vi "Run_Expand_Constraints_decomposition.vi"() -> (0 "constraints cluster":T1)   [LabVIEW 2015]
uses:
  <vilib>/Utility/file.llb/Read Delimited Spreadsheet (DBL).vi
panel:
  in  "Lq":i32=15
  out "OmegaChain":dbl[](array[numeric])
  out "beta":dbl[](array[numeric])
  out "gamma":dbl
  out "weight":dbl
  in  "w0":dbl=100000.0
  out "Nc":i32
  out "one constraint":dbl[](array[numeric])
  out "size(s)":i32[](array[numeric])
  out "all constraints":dbl[][](array[numeric])
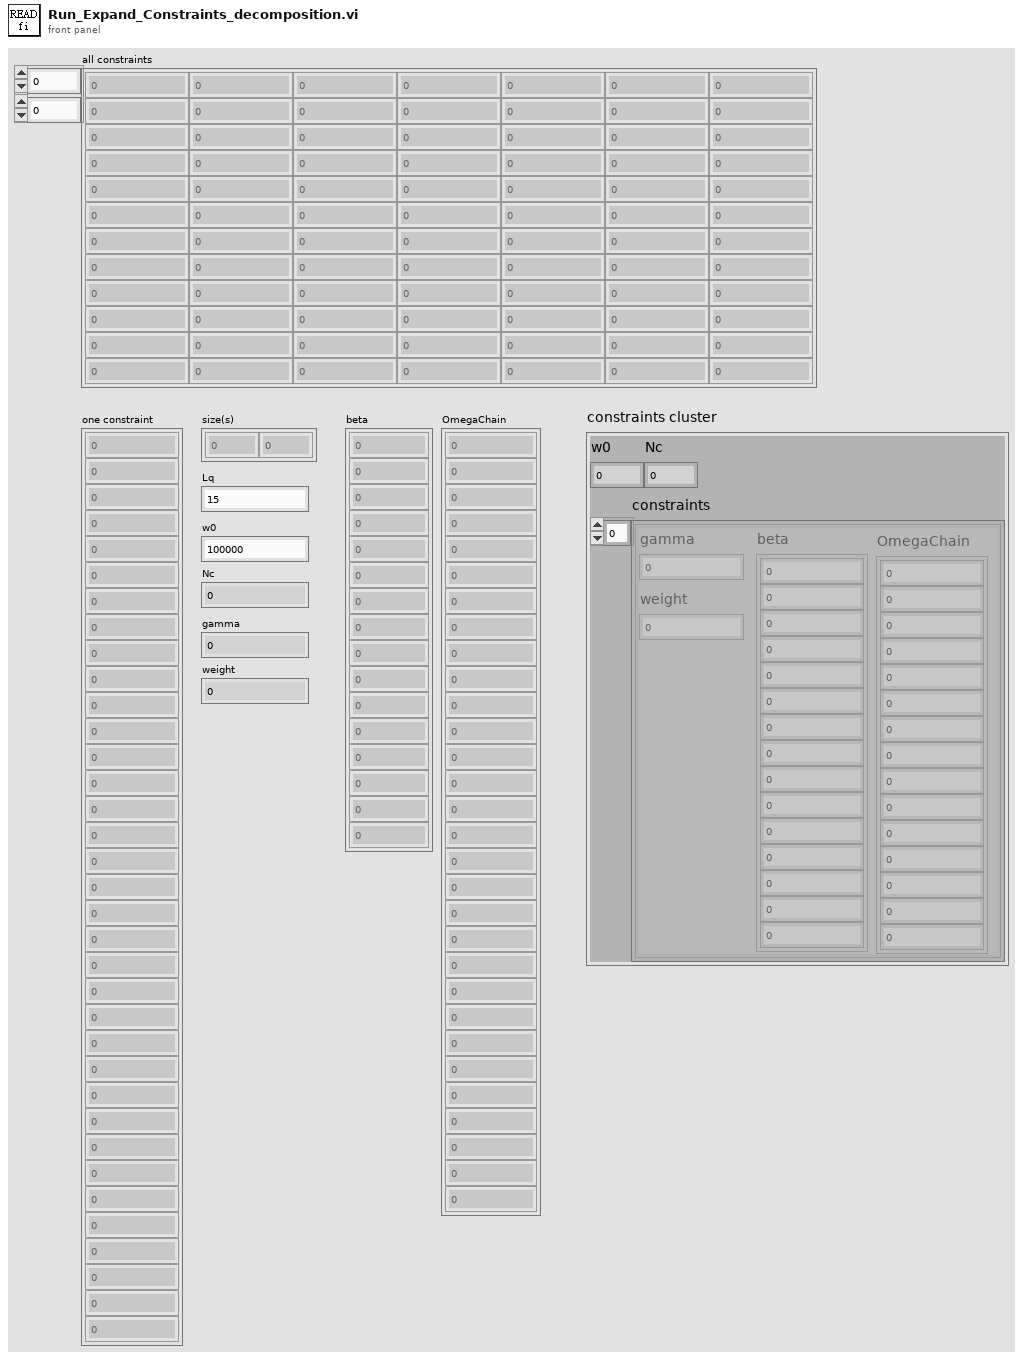
[diagram p1: front panel]
types:
  T1 = cluster{"w0":dbl, "constraints":cluster{"beta":dbl[], "gamma":dbl, "OmegaChain":dbl[], "weight":dbl}[], "Nc":i32}
  T2 = cluster{"beta":dbl[], "gamma":dbl, "OmegaChain":dbl[], "weight":dbl}
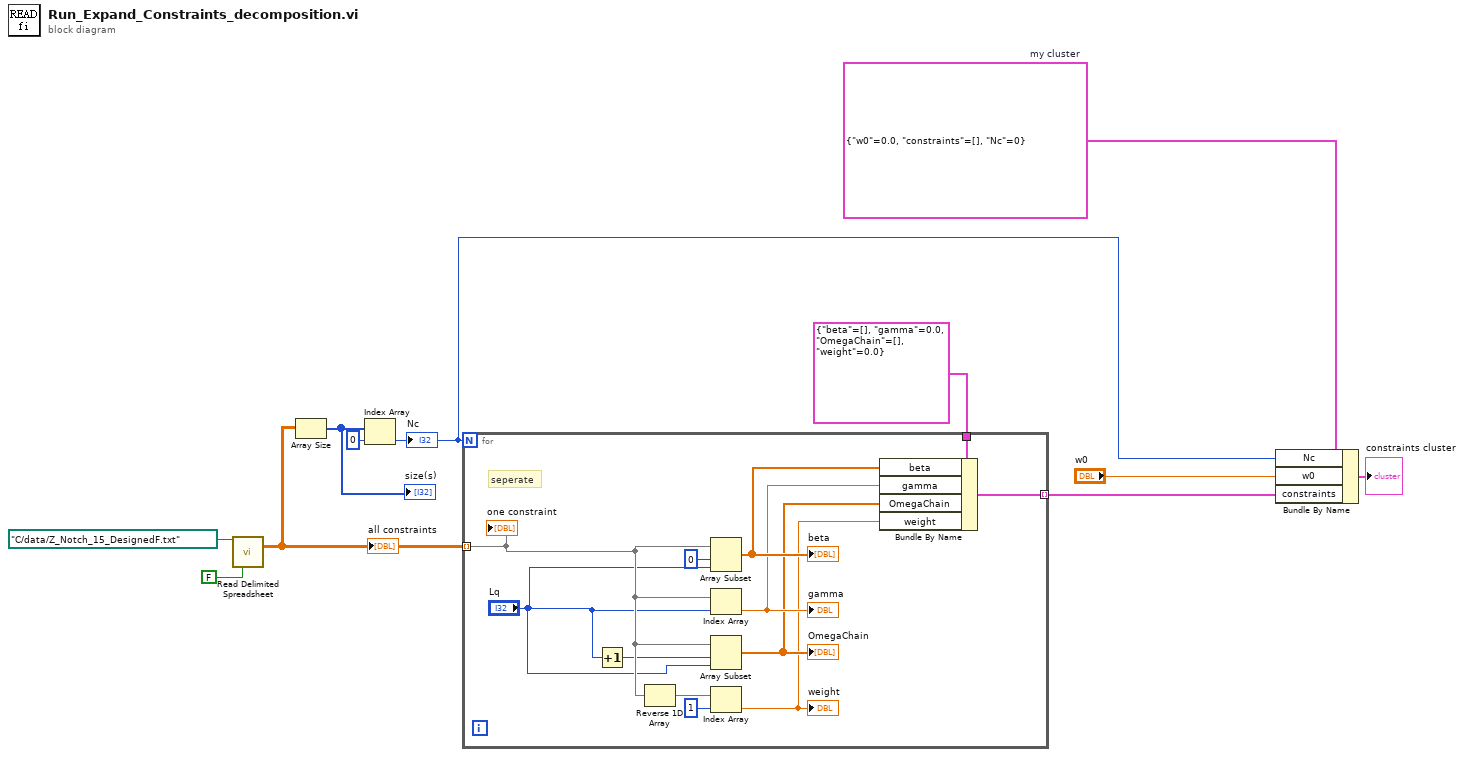
[diagram p0: block diagram]
diagram:
  w6 = T1 {"w0"=0.0, "constraints"=[], "Nc"=0}  # my cluster
  n1 = call-poly <vilib>:"Read Delimited Spreadsheet.vi"("file path (dialog if empty)"=path "C:/data/Z_Notch_15_DesignedF.txt", "transpose? (F)"=FALSE) -> ("all rows"=w8:dbl[][])  [unwired: 8 in, 5 out]
  "all constraints" <- w8
  n2 = Array Size(array=w8) -> (size(s)=w10:i32[])
  "size(s)" <- w10
  n3 = Index Array(array=w10, index=0) -> (element=w4:i32)
  "Nc" <- w4
  n4 = for {
    N: w4 -> [_]
    tunnel: w8 -> [w23] mode=indexing
    tunnel: [w13] -> w5 mode=indexing
    tunnel: T2 {"beta"=[], "gamma"=0.0, "OmegaChain"=[], "weight"=0.0} -> [w18]
    # "seperate"
    n5 = Increment(x="Lq") -> (x+1=w21:i32)
    n6 = Reverse 1D Array(array=w23) -> (reversed array=w20:dbl[])
    n7 = Array Subset(array=w23, index=0, length="Lq") -> (w17:dbl[])
    "beta" <- w17
    n8 = Index Array(array=w23, index="Lq") -> (element=w16:dbl)
    "gamma" <- w16
    n9 = Array Subset(array=w23, index=w21, length="Lq") -> (w15:dbl[])
    "OmegaChain" <- w15
    n10 = Index Array(array=w20, index=1) -> (element=w14:dbl)
    "weight" <- w14
    n11 = Bundle By Name(cluster=w18, "beta"=w17, "gamma"=w16, "OmegaChain"=w15, "weight"=w14) -> (w13:T2)
    "one constraint" <- w23
  }
  n12 = Bundle By Name(cluster=w6, "Nc"=w4, "w0"="w0", "constraints"=w5) -> (→"constraints cluster":T1)
